vi "Sub00_Setup.vi"(7 "Enum":T1(ring), 8 "error in (no error)":errorcluster, 9 "Tab Control":T2(tab), 10 "Select sequence":string(combo)="F1", 11 "Path":path) -> (0 "error out":errorcluster, 1 "filenames":string[](array[string]), 2 "name":string, 3 "path out":path)   [LabVIEW 2019]
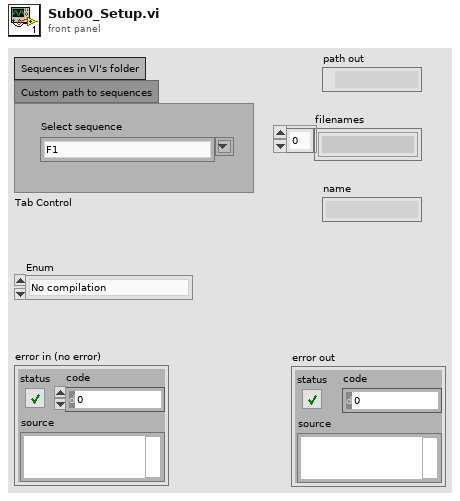
[diagram p1: front panel]
types:
  T1 = enum16{"No compilation", "No memory", "With memory"}
  T2 = enum32{"Sequences in VI's folder", "Custom path to sequences"}
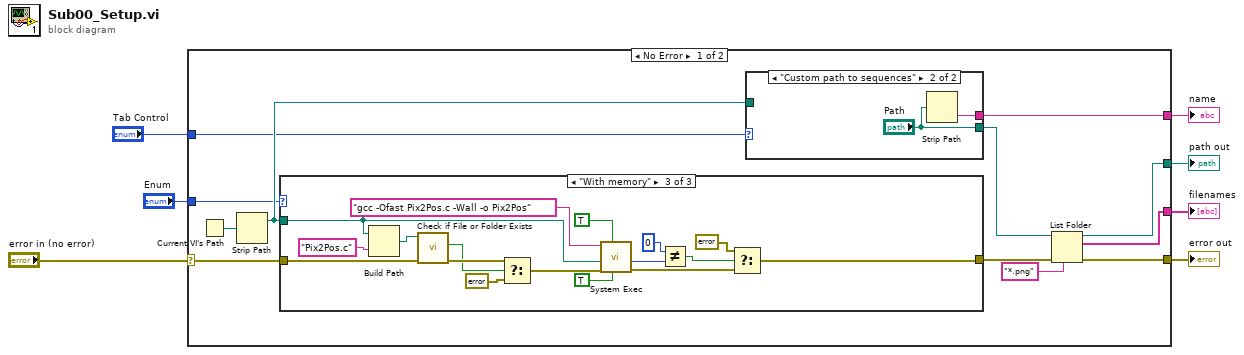
[diagram p0: block diagram]
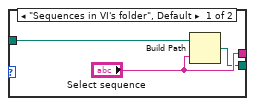
[diagram p2: hidden frame]
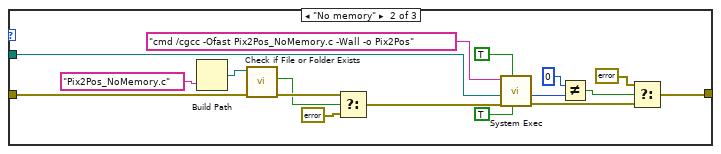
[diagram p4: hidden frame]
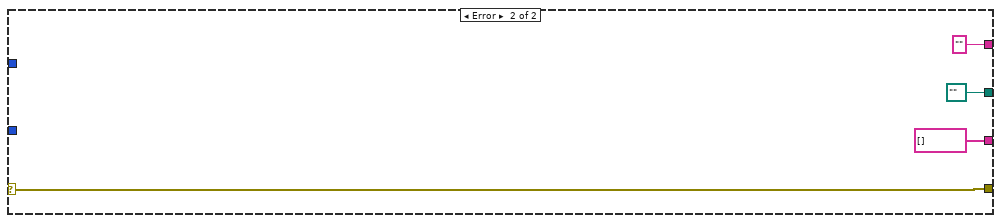
[diagram p5: hidden frame]
diagram:
  n1 = case shown="No Error" "error in (no error)" {
    selector: "error in (no error)" -> [w8 w60]
    tunnel: [w15 w60] -> w7
    tunnel: [w14 path "" ("path out")] -> w6
    tunnel: [w13 string[] [] ("filenames")] -> w5
    tunnel: [w11 "" ("name")] -> w4
    tunnel: "Enum" -> [w10 _]
    tunnel: "Tab Control" -> [w9 _]
    frame No Error {
      n2 = Current VI's Path() -> (path=w18:path)
      n3 = Strip Path(path=w18) -> (stripped path=w19:path)  [unwired: 1 out]
      n4 = case shown="\"With memory\"" w10 {
        tunnel: w19 -> [_ w42 w48]
        tunnel: w8 -> [w25 w27 w50]
        tunnel: [w25 w34 w52] -> w16
        frame "No compilation", Default {
        }
        frame "No memory" {
          n5 = Build Path(name or relative path="Pix2Pos_NoMemory.c") -> (appended path=w32:path)  [unwired: 1 in]
          n6 = call <vilib>:"Check if File or Folder Exists.vi"("error in (no error)"=w27, "path"=w32) -> ("error out"=w30:errorcluster, "file or folder exists?"=w29:bool)  [unwired: 7 in, 1 out]
          n7 = Select(t=w30, s=w29, f=errorcluster {"status"=TRUE, "code"=11, "source"="Pix2Pos_NoMemory.c doesn't exist"} ("t")) -> (s? t:f=w26:errorcluster)
          n8 = call <vilib>:"System Exec.vi"("run minimized? (F)"=TRUE, "wait until completion? (T)"=TRUE, "error in (no error)"=w26, "working directory"=w42, "command line"="cmd /cgcc -Ofast Pix2Pos_NoMemory.c -Wall -o Pix2Pos") -> ("error out"=w35:errorcluster, "return code"=w39:i32)  [unwired: 3 in, 2 out]
          n9 = Not Equal?(x=0 ("y"), y=w39) -> (x != y?=w36:bool)
          n10 = Select(t=errorcluster {"status"=TRUE, "code"=11, "source"="Compilation failed"}, s=w36, f=w35) -> (s? t:f=w34:errorcluster)
        }
        frame "With memory" {
          n11 = Build Path(base path=w48, name or relative path="Pix2Pos.c") -> (appended path=w49:path)
          n12 = call <vilib>:"Check if File or Folder Exists.vi"("error in (no error)"=w50, "path"=w49) -> ("error out"=w46:errorcluster, "file or folder exists?"=w45:bool)  [unwired: 7 in, 1 out]
          n13 = Select(t=w46, s=w45, f=errorcluster {"status"=TRUE, "code"=11, "source"="Pix2Pos.c doesn't exist"} ("t")) -> (s? t:f=w44:errorcluster)
          n14 = call <vilib>:"System Exec.vi"("run minimized? (F)"=TRUE, "wait until completion? (T)"=TRUE, "error in (no error)"=w44, "working directory"=w48, "command line"="gcc -Ofast Pix2Pos.c -Wall -o Pix2Pos") -> ("error out"=w53:errorcluster, "return code"=w57:i32)  [unwired: 3 in, 2 out]
          n15 = Not Equal?(x=0 ("y"), y=w57) -> (x != y?=w54:bool)
          n16 = Select(t=errorcluster {"status"=TRUE, "code"=11, "source"="Compilation failed"}, s=w54, f=w53) -> (s? t:f=w52:errorcluster)
        }
      }
      n17 = case shown="\"Custom path to sequences\"" w9 {
        tunnel: ["Select sequence" w23] -> w11
        tunnel: w19 -> [w21 _]
        tunnel: [w20 "Path"] -> w17
        frame "Sequences in VI's folder", Default {
          n18 = Build Path(base path=w21, name or relative path="Select sequence") -> (appended path=w20:path)
        }
        frame "Custom path to sequences" {
          n19 = Strip Path(path="Path") -> (name=w23:string)  [unwired: 1 out]
        }
      }
      n20 = List Folder(path=w17, pattern="*.png", error in=w16) -> (path out=w14:path, filenames=w13:string[], error out=w15:errorcluster)  [unwired: 1 in, 1 out]
    }
    frame Error {
    }
  }
  "error out" <- w7
  "path out" <- w6
  "filenames" <- w5
  "name" <- w4
